vi "SetMarquee_Video.vi"(4 "opacity":i32=255, 5 "y-coordinate":i32=10, 6 "x-coordinate":i32=255, 7 "error in (no error)":errorcluster, 8 "String":string, 10 "VLC Variables":T1) -> (0 "error out":errorcluster)   [LabVIEW 2012]
doc: "Show a given string in a given x,y coordinates with a given opacity inside the video"
uses:
  Controls-Webcam/VLC Var.ctl
panel:
  in  "libvlc.dll path":path=path "C:/Users/npueyo/Desktop/VLC Video/VLC Portable/App/vlc/libvlc.dll"
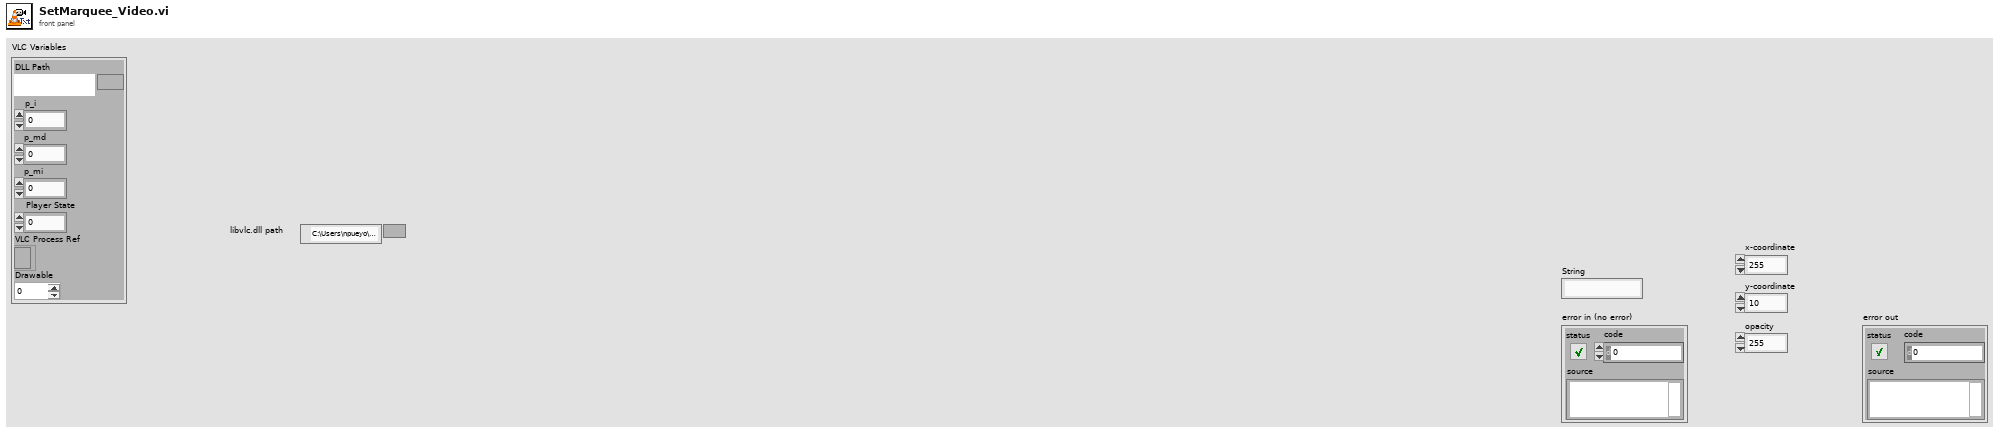
[diagram p1: front panel]
types:
  T1 = typedef "VLC Var.ctl" = cluster{"DLL Path":path, "p_i":i32, "p_md":i32, "p_mi":i32, "Player State":i32, "VLC Process Ref":refnum<k24>, "Drawable":i32}
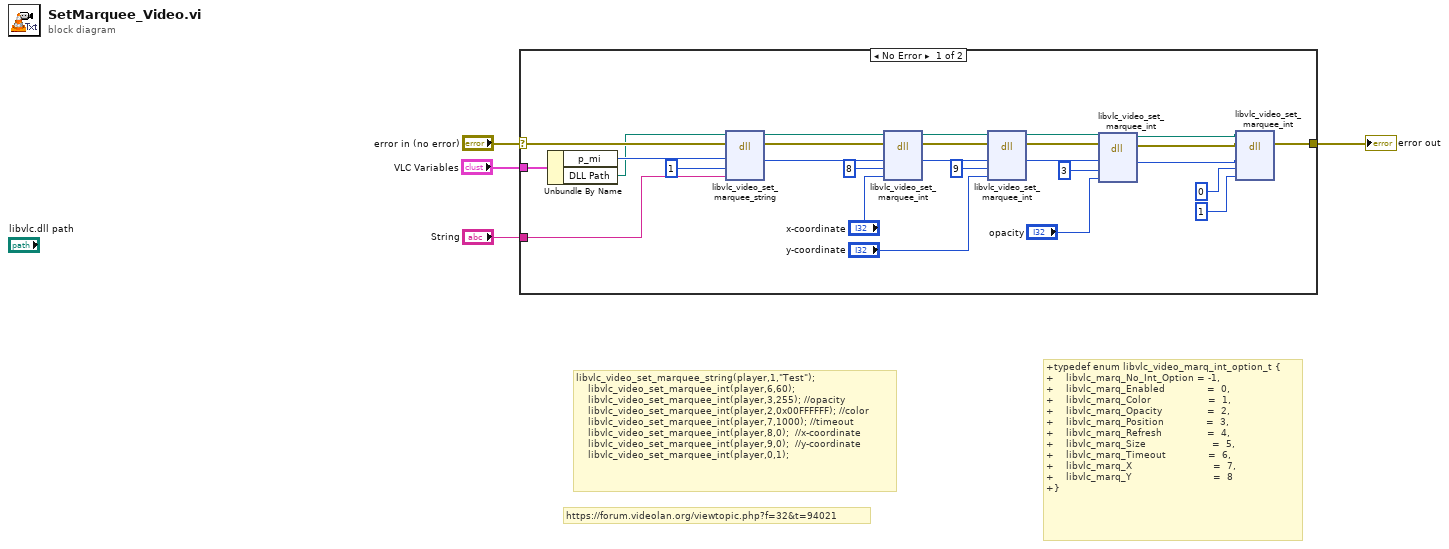
[diagram p0: block diagram]
diagram:
  # "https://forum.videolan.org/viewtopic.php?f=32&t=94021"
  # "libvlc_video_set_marquee_string(player,1,\"Test\");\n    libvlc_video_set_marquee_int(player,6,60);\n    libvlc_video_set_marquee_int(player,3,255); //opacity\n    libvlc_video_set_marquee_int(player,2,0x00FFFFFF); //color\n    libvlc_video_set_marquee_int(player,7,1000); //timeout\n    libvlc_video_set_marquee_int(player,8,0);  //x-coordinate\n    libvlc_video_set_marquee_int(player,9,0);  //y-coordinate\n    libvlc_video_set_marquee_int(player,0,1);"
  # "+typedef enum libvlc_video_marq_int_option_t {\n+    libvlc_marq_No_Int_Option = -1,\n+    libvlc_marq_Enabled              =  0,\n+    libvlc_marq_Color                   =  1,\n+    libvlc_marq_Opacity               =  2,\n+    libvlc_marq_Position              =  3,\n+    libvlc_marq_Refresh               =  4,\n+    libvlc_marq_Size                      =  5,\n+    libvlc_marq_Timeout              =  6,\n+    libvlc_marq_X                           =  7,\n+    libvlc_marq_Y                           =  8\n+}"
  n1 = case shown="No Error" "error in (no error)" {
    selector: "error in (no error)" -> [w6 w32]
    tunnel: [w31 w32] -> w4
    tunnel: "String" -> [w30 _]
    tunnel: "VLC Variables" -> [w8 _]
    frame No Error {
      n2 = Unbundle By Name(w8) -> ("p_mi"=w7:i32, "DLL Path"=w5:path)
      n3 = dll-call lib="C:/Program Files (x86)/VideoLAN/VLC/libvlc.dll" fn="libvlc_video_set_marquee_string"(path in=w5, error in=w6, "p_mi"=w7, "option"=u32 1, "psz_text"=w30) -> (path out=w25:path, error out=w26:errorcluster, "p_mi"=w29:i32)  [unwired: 4 in]
      n4 = dll-call lib="C:/Program Files (x86)/VideoLAN/VLC/libvlc.dll" fn="libvlc_video_set_marquee_int"(path in=w25, error in=w26, "p_mi"=w29, "option"=u32 8, "i_val"="x-coordinate") -> (path out=w27:path, error out=w9:errorcluster, "p_mi"=w28:i32)  [unwired: 4 in]
      n5 = dll-call lib="C:/Program Files (x86)/VideoLAN/VLC/libvlc.dll" fn="libvlc_video_set_marquee_int"(path in=w27, error in=w9, "p_mi"=w28, "option"=u32 9, "i_val"="y-coordinate") -> (path out=w13:path, error out=w14:errorcluster, "p_mi"=w15:i32)  [unwired: 4 in]
      n6 = dll-call lib="C:/Program Files (x86)/VideoLAN/VLC/libvlc.dll" fn="libvlc_video_set_marquee_int"(path in=w13, error in=w14, "p_mi"=w15, "option"=u32 3, "i_val"="opacity") -> (path out=w12:path, error out=w11:errorcluster, "p_mi"=w10:i32)  [unwired: 4 in]
      n7 = dll-call lib="C:/Program Files (x86)/VideoLAN/VLC/libvlc.dll" fn="libvlc_video_set_marquee_int"(path in=w12, error in=w11, "p_mi"=w10, "option"=u32 0, "i_val"=1) -> (error out=w31:errorcluster)  [unwired: 5 in, 1 out]
    }
    frame Error {
    }
  }
  "error out" <- w4
